vi "Disconnect Network Resource.vi"(8 "error in (no error)":errorcluster, 10 "force disconnect (T)":bool=TRUE, 11 "name":string) -> (0 "error out":errorcluster)   [LabVIEW 2023, in "WINNET.lvlib"]
doc: "This VI will disconnect the local machine from a network drive or printer (e.g. F: or LPT3). If the \"force disconnect\" input is FALSE and open files or print jobs on the specified resource exist, error 49 is returned (WN_OPEN_FILES)."
uses:
  WINNET.lvlib
  MPR.DLL
panel:
  out "errors":u16(ring) items=["WN_SUCCESS", "WN_NOT_SUPPORTED", "WN_NET_ERROR", "WN_MORE_DATA", "WN_BAD_POINTER", "WN_BAD_VALUE", "WN_BAD_PASSWORD", "WN_ACCESS_DENIED", "WN_FUNCTION_BUSY", "WN_WINDOWS_ERROR", "WN_BAD_USER", "WN_OUT_OF_MEMORY", "WN_CANCEL", "WN_CONTINUE", "WN_OPEN_FILES"]
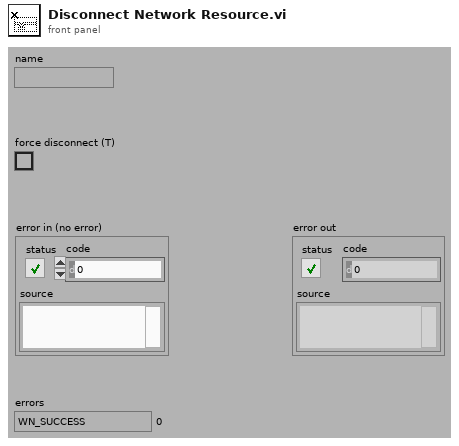
[diagram p1: front panel]
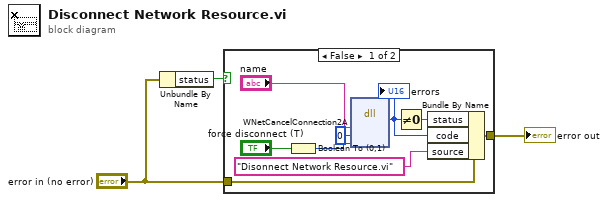
[diagram p0: block diagram]
diagram:
  n1 = Unbundle By Name("error in (no error)") -> ("status"=w3:bool)
  n2 = case shown="False" w3 {
    tunnel: "error in (no error)" -> [w7 w13]
    tunnel: [w6 w13] -> w1
    frame False {
      n3 = Boolean To (0,1)(Boolean="force disconnect (T)") -> (0, 1=w5:i16)
      n4 = dll-call lib="MPR.DLL" fn="WNetCancelConnection2A"("lpszName"="name", "dwFlags"=u32 0, "fForce"=w5) -> ("ReturnVal"=w9:u32)  [unwired: 5 in, 3 out]
      "errors" <- w9
      n5 = Not Equal To 0?(x=w9) -> (x != 0?=w10:bool)
      n6 = Bundle By Name(cluster=w7, "status"=w10, "code"=w9, "source"="Disonnect Network Resource.vi") -> (w6:errorcluster)
    }
    frame True {
    }
  }
  "error out" <- w1
